vi "SS2 Live_Settings Q.vi"() -> (5 "error out":errorcluster, 7 "Queue out":refnum<queue>)   [LabVIEW 2019]
uses:
  SS2 Live_Settings Q Element.ctl
  SS2 Live_Settings Q Action.ctl
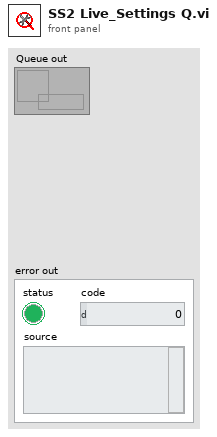
[diagram p1: front panel]
types:
  T1 = typedef "SS2 Live_Settings Q Element.ctl" = cluster{"Action":T2, "Data":variant}
  T2 = typedef "SS2 Live_Settings Q Action.ctl" = enum16{"Idle", "Store Current Configuration", "Rename Current Configuration", "Delete Current Configuration", "Update Image ROI Information", "Quit"}
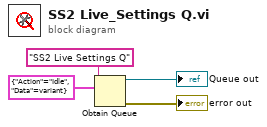
[diagram p0: block diagram]
diagram:
  n1 = Obtain Queue(name (unnamed)="SS2 Live Settings Q", element data type=T1 {"Action"=enum."Idle", "Data"=variant} ("Settings Q Element")) -> (queue out=→"Queue out":refnum<queue>, error out=→"error out":errorcluster)  [unwired: 3 in, 1 out]
